vi "Center alignment.vi"(9 "위치:위쪽":i32, 10 "참조":refnum<vi>, 11 "VI 입력":refnum<vi>) -> (0 "에러 출력":errorcluster, 3 "Bounds":cluster{"Width":u32, "Height":u32})   [LabVIEW 2019]
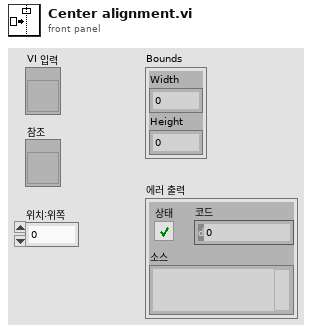
[diagram p1: front panel]
types:
  T1 = typedef "LVRectTypeDef.ctl" = cluster{"Left":i16, "Top":i16, "Right":i16, "Bottom":i16}
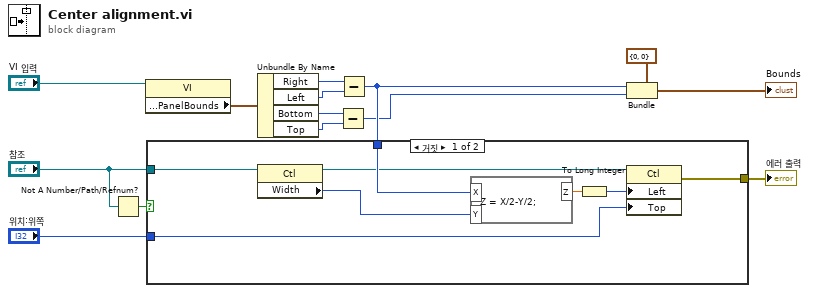
[diagram p0: block diagram]
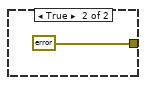
[diagram p2: hidden frame]
diagram:
  n1 = Not A Number/Path/Refnum?(number/path/refnum="참조") -> (NaN/Path/Refnum?=w1:bool)
  n2 = property class="VI"(reference="VI 입력") -> ("Front Panel.PanelBounds"=w5:T1)  [unwired: 1 in, 2 out]
  n3 = Unbundle By Name(w5) -> ("Right"=w6:i16, "Left"=w7:i16, "Bottom"=w8:i16, "Top"=w9:i16)
  n4 = Subtract(x=w8, y=w9) -> (x-y=w10:i16)
  n5 = Subtract(x=w6, y=w7) -> (x-y=w13:i16)
  n6 = case shown="거짓" w1 {
    tunnel: w13 -> [w21 _]
    tunnel: "위치:위쪽" -> [w18 _]
    tunnel: "참조" -> [w17 _]
    tunnel: [w15 errorcluster {"status"=FALSE, "code"=0, "source"=""} ("에러 출력")] -> w3
    frame False {
      n7 = property on="프로퍼티 노드" class="Ctl"(reference=w17) -> ("Width"=w19:u32)  [unwired: 1 in, 2 out]
      n8 = formula code="Z = X/2-Y/2;"("X"=w21, "Y"=w19) -> ("Z"=w20:dbl)
      n9 = To Long Integer(number=w20) -> (32bit integer=w16:i32)
      n10 = property on="프로퍼티 노드" class="Ctl"(reference=w17, "Left"=w16, "Top"=w18) -> (error out=w15:errorcluster)  [unwired: 1 in, 1 out]
    }
    frame True {
    }
  }
  "에러 출력" <- w3
  n11 = Bundle(cluster=cluster{"Width":u32, "Height":u32} {"Width"=0, "Height"=0} ("Bounds"), "Width"=w13, "Height"=w10) -> (→"Bounds":cluster{"Width":u32, "Height":u32})
